vi "Read Acquisition  Enqueuer.vi"(8 "error in (no error)":errorcluster, 11 "Grayscale in":refnum<class "Grayscale.lvclass">) -> (0 "error out":errorcluster, 2 "Actor Framework:Message Enqueuer":refnum<class "Message Enqueuer.lvclass">, 3 "Grayscale out":refnum<class "Grayscale.lvclass">)   [LabVIEW 2015, in "Tests.lvlib" / "Grayscale.lvclass"]
uses:
  Grayscale.lvclass
  <vilib>/ActorFramework/Message Enqueuer/Message Enqueuer.lvclass
  Grayscale.lvclass/Grayscale.ctl
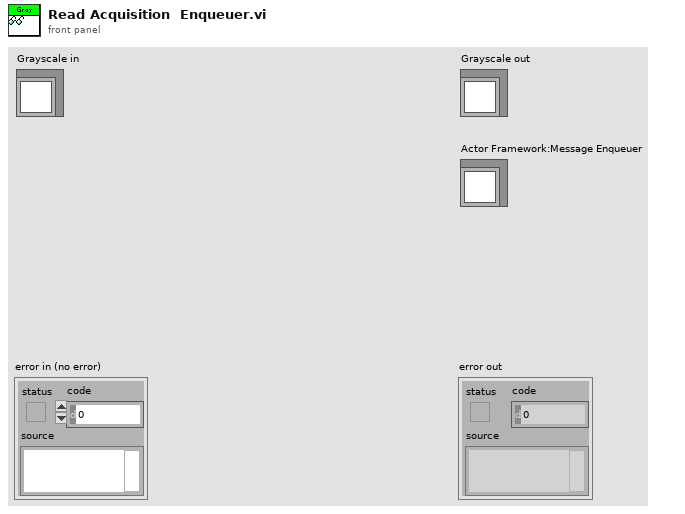
[diagram p1: front panel]
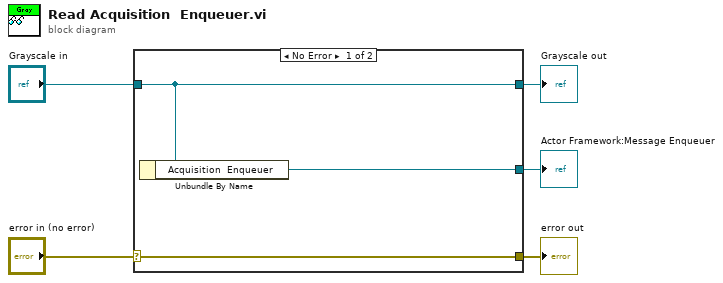
[diagram p0: block diagram]
diagram:
  n1 = case shown="No Error" "error in (no error)" {
    selector: "error in (no error)" -> [w8 w9]
    tunnel: [w8 w9] -> w4
    tunnel: [w7 w10] -> w2
    tunnel: "Grayscale in" -> [w7 w10]
    tunnel: [w6 _] -> w1
    frame No Error {
      n2 = Unbundle By Name(w7) -> ("Acquisition  Enqueuer"=w6:refnum<class "Message Enqueuer.lvclass">)
    }
    frame Error {
    }
  }
  "error out" <- w4
  "Grayscale out" <- w2
  "Actor Framework:Message Enqueuer" <- w1
